vi "set AC test parameters.vi"(7 "AC Parameters":T1={"Voltage Level [V] "=1500, "Hi Limit [A]"=0.005, "Test Time [s] "=3.3, "Lo Limit [A]"=0.001, "ARC Limit [A]"=0.005, "Ramp Time [s] "=1.1, "Fall Time [s]"=2.2} {"Voltage Level [V]" format="%.3p"; "Hi Limit [A]" format="%#_6p"; "Lo Limit [A]" format="%#_6p"; "ARC Limit [A]" format="%#_6p"}, 8 "error in (no error)":errorcluster, 10 "Step":T2 min=1 max=99 step=1, 11 "VISA Refnum in":refnum<visa-resource-name>) -> (0 "error out":errorcluster, 3 "VISA Refnum out":refnum<visa-resource-name>)   [LabVIEW 2025]
uses:
  Type Def/steps--ring.ctl
  Type Def/AC-DC modes--ring.ctl
  Type Def/AC-DC-IR modes--ring.ctl
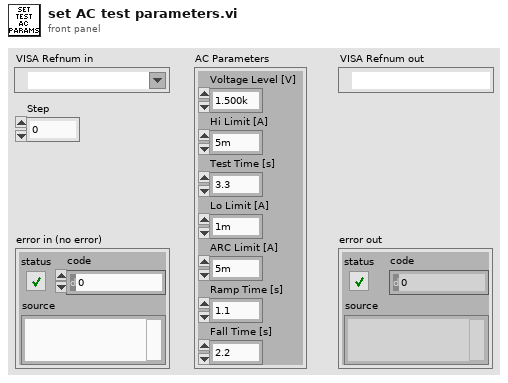
[diagram p1: front panel]
types:
  T1 = cluster{"Voltage Level [V] ":u16, "Hi Limit [A]":dbl, "Test Time [s] ":dbl, "Lo Limit [A]":dbl, "ARC Limit [A]":dbl, "Ramp Time [s] ":dbl, "Fall Time [s]":dbl}
  T2 = typedef "steps--ring.ctl" = u8
  T3 = typedef "AC-DC modes--ring.ctl" = i32
  T4 = typedef "AC-DC-IR modes--ring.ctl" = u16
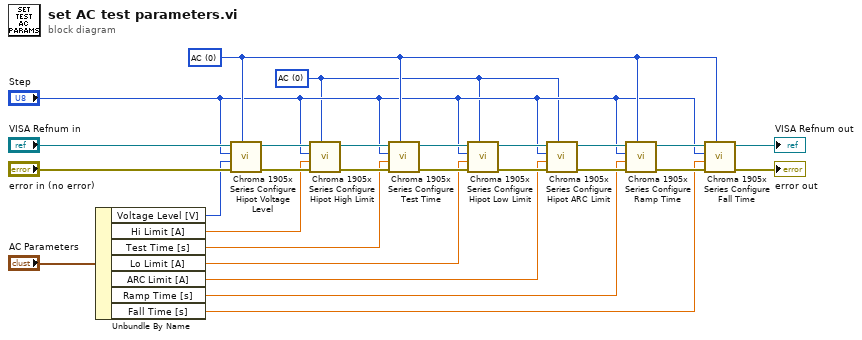
[diagram p0: block diagram]
diagram:
  w9 = T3 0 items=["AC", "DC"] ("Mode")
  w13 = T4 0 items=["AC", "DC", "IR"] ("Mode")
  n1 = Unbundle By Name("AC Parameters") -> ("Voltage Level [V]"=w7:u16, "Hi Limit [A]"=w6:dbl, "Test Time [s]"=w5:dbl, "Lo Limit [A]"=w4:dbl, "ARC Limit [A]"=w3:dbl, "Ramp Time [s]"=w2:dbl, "Fall Time [s]"=w1:dbl)
  n2 = call "Chroma 1905x Series Configure Hipot Voltage Level.vi"("Mode"=w13, "error in (no error)"="error in (no error)", "Voltage Level [V]"=w7, "Step"="Step", "VISA resource name"="VISA Refnum in") -> ("error out"=w19:errorcluster, "VISA resource name out"=w16:refnum<visa-resource-name>)  [unwired: 5 in]
  n3 = call "Chroma 1905x Series Configure Hipot High Limit.vi"("Mode"=w9, "error in (no error)"=w19, "Hi Limit [A]"=w6, "Step"="Step", "VISA resource name"=w16) -> ("error out"=w26:errorcluster, "VISA resource name out"=w27:refnum<visa-resource-name>)  [unwired: 5 in]
  n4 = call "Chroma 1905x Series Configure Test Time.vi"("Mode"=w13, "error in (no error)"=w26, "Test Time [s]"=w5, "Step"="Step", "VISA resource name"=w27) -> ("error out"=w15:errorcluster, "VISA resource name out"=w14:refnum<visa-resource-name>)  [unwired: 5 in]
  n5 = call "Chroma 1905x Series Configure Hipot Low Limit.vi"("Mode"=w9, "error in (no error)"=w15, "Lo Limit [A]"=w4, "Step"="Step", "VISA resource name"=w14) -> ("error out"=w20:errorcluster, "VISA resource name out"=w21:refnum<visa-resource-name>)  [unwired: 5 in]
  n6 = call "Chroma 1905x Series Configure Hipot ARC Limit.vi"("Mode"=w9, "error in (no error)"=w20, "ARC Limit [A]"=w3, "Step"="Step", "VISA resource name"=w21) -> ("error out"=w22:errorcluster, "VISA resource name out"=w24:refnum<visa-resource-name>)  [unwired: 5 in]
  n7 = call "Chroma 1905x Series Configure Ramp Time.vi"("Mode"=w13, "error in (no error)"=w22, "Ramp Time [s]"=w2, "Step"="Step", "VISA resource name"=w24) -> ("error out"=w23:errorcluster, "VISA resource name out"=w25:refnum<visa-resource-name>)  [unwired: 5 in]
  n8 = call "Chroma 1905x Series Configure Fall Time.vi"("Mode"=w13, "error in (no error)"=w23, "Fall Time [s]"=w1, "Step"="Step", "VISA resource name"=w25) -> ("error out"=→"error out":errorcluster, "VISA resource name out"=→"VISA Refnum out":refnum<visa-resource-name>)  [unwired: 5 in]
